vi "Read CCDF (Reference Trace).vi"(8 "error in (no error)":errorcluster, 11 "VISA resource name":refnum<visa-resource-name>) -> (0 "error out":errorcluster, 1 "Average Power Data":dbl, 2 "Max X-axis Value (dB)":dbl, 3 "VISA resource name out":refnum<visa-resource-name>, 4 "Peak-to-average Data":dbl, 5 "Peak Power Data":dbl, 6 "Reference Trace Data":dbl[](array[numeric]))   [LabVIEW 2014, in "Agilent U2000 Series.lvlib"]
doc: "Retrieves the CCDF reference trace data.\n\nNote: \nIf there was no previously saved trace, error C221, \"Settings conflict\" occurs. You need to check the status of the saved reference trace using PST:CCDF:STOR:REF?.\nThis VI is not applicable for U2040 X-Series."
uses:
  Agilent U2000 Series.lvlib
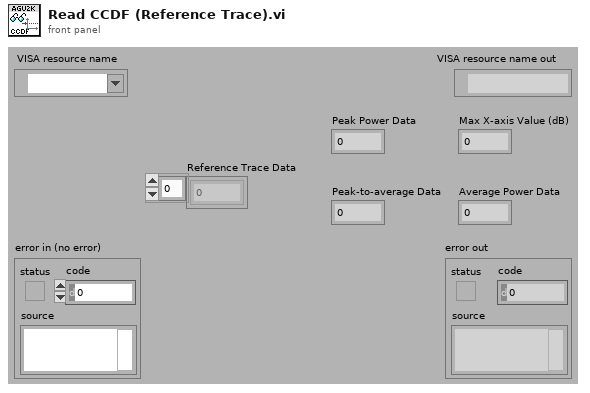
[diagram p1: front panel]
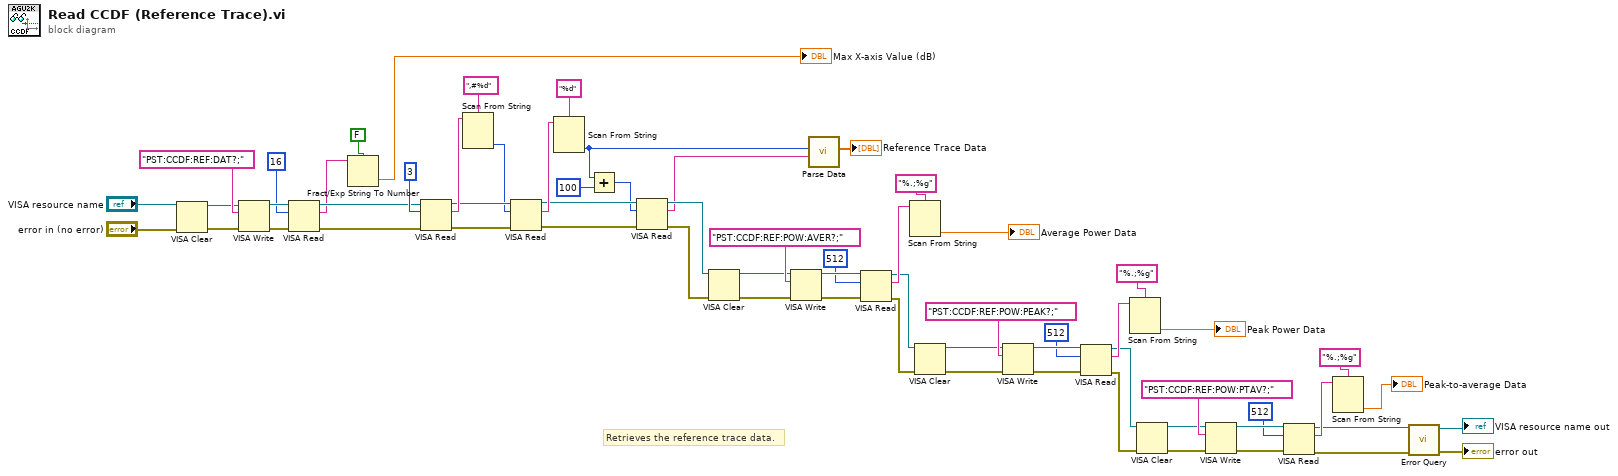
[diagram p0: block diagram]
diagram:
  # "Retrieves the reference trace data."
  n1 = VISA Clear(VISA resource name="VISA resource name", error in (no error)="error in (no error)") -> (VISA resource name out=w43:refnum<visa-resource-name>, error out=w42:errorcluster)
  n2 = VISA Write(VISA resource name=w43, write buffer="PST:CCDF:REF:DAT?;", error in (no error)=w42) -> (VISA resource name out=w17:refnum<visa-resource-name>, error out=w16:errorcluster)  [unwired: 1 out]
  n3 = VISA Read(VISA resource name=w17, byte count=u32 16, error in (no error)=w16) -> (VISA resource name out=w14:refnum<visa-resource-name>, read buffer=w12:string, error out=w13:errorcluster)  [unwired: 1 out]
  n4 = Fract/Exp String To Number(use system decimal point (T)=FALSE, string=w12) -> (number=→"Max X-axis Value (dB)":dbl)  [unwired: 3 out]
  n5 = VISA Read(VISA resource name=w14, byte count=u32 3, error in (no error)=w13) -> (VISA resource name out=w28:refnum<visa-resource-name>, read buffer=w30:string, error out=w27:errorcluster)  [unwired: 1 out]
  n6 = Scan From String(format string=",#%d", input string=w30) -> (output 1=w26:i32)  [unwired: 2 in, 4 out]
  n7 = VISA Read(VISA resource name=w28, byte count=w26, error in (no error)=w27) -> (VISA resource name out=w23:refnum<visa-resource-name>, read buffer=w24:string, error out=w22:errorcluster)  [unwired: 1 out]
  n8 = Scan From String(format string="%d", input string=w24) -> (output 1=w4:i32)  [unwired: 2 in, 4 out]
  n9 = Add(x=w4, y=100) -> (x+y=w20:i32)
  n10 = VISA Read(VISA resource name=w23, byte count=w20, error in (no error)=w22) -> (VISA resource name out=w19:refnum<visa-resource-name>, read buffer=w3:string, error out=w18:errorcluster)  [unwired: 1 out]
  n11 = VISA Clear(VISA resource name=w19, error in (no error)=w18) -> (VISA resource name out=w40:refnum<visa-resource-name>, error out=w41:errorcluster)
  n12 = VISA Write(VISA resource name=w40, write buffer="PST:CCDF:REF:POW:AVER?;", error in (no error)=w41) -> (VISA resource name out=w64:refnum<visa-resource-name>, error out=w63:errorcluster)  [unwired: 1 out]
  n13 = call "Parse Data.vi"("Read Buffer"=w3, "Data Length"=w4) -> ("Output Data Array"=→"Reference Trace Data":dbl[])  [unwired: 9 out]
  n14 = VISA Read(VISA resource name=w64, byte count=u32 512, error in (no error)=w63) -> (VISA resource name out=w37:refnum<visa-resource-name>, read buffer=w61:string, error out=w36:errorcluster)  [unwired: 1 out]
  n15 = Scan From String(format string="%.;%g", input string=w61) -> (output 1=→"Average Power Data":dbl)  [unwired: 2 in, 4 out]
  n16 = VISA Clear(VISA resource name=w37, error in (no error)=w36) -> (VISA resource name out=w39:refnum<visa-resource-name>, error out=w38:errorcluster)
  n17 = VISA Write(VISA resource name=w39, write buffer="PST:CCDF:REF:POW:PEAK?;", error in (no error)=w38) -> (VISA resource name out=w57:refnum<visa-resource-name>, error out=w56:errorcluster)  [unwired: 1 out]
  n18 = VISA Read(VISA resource name=w57, byte count=u32 512, error in (no error)=w56) -> (VISA resource name out=w33:refnum<visa-resource-name>, read buffer=w54:string, error out=w34:errorcluster)  [unwired: 1 out]
  n19 = Scan From String(format string="%.;%g", input string=w54) -> (output 1=→"Peak Power Data":dbl)  [unwired: 2 in, 4 out]
  n20 = VISA Clear(VISA resource name=w33, error in (no error)=w34) -> (VISA resource name out=w32:refnum<visa-resource-name>, error out=w35:errorcluster)
  n21 = VISA Write(VISA resource name=w32, write buffer="PST:CCDF:REF:POW:PTAV?;", error in (no error)=w35) -> (VISA resource name out=w50:refnum<visa-resource-name>, error out=w49:errorcluster)  [unwired: 1 out]
  n22 = VISA Read(VISA resource name=w50, byte count=u32 512, error in (no error)=w49) -> (VISA resource name out=w8:refnum<visa-resource-name>, read buffer=w47:string, error out=w5:errorcluster)  [unwired: 1 out]
  n23 = Scan From String(format string="%.;%g", input string=w47) -> (output 1=→"Peak-to-average Data":dbl)  [unwired: 2 in, 4 out]
  n24 = call "Error Query.vi"("error in (no error)"=w5, "VISA resource name"=w8) -> ("error out"=→"error out":errorcluster, "VISA resource name out"=→"VISA resource name out":refnum<visa-resource-name>)  [unwired: 8 out]
